vi "Joystick 1 Button Handler.vi"(8 "error in (no error)":errorcluster, 11 "Buttons":bool[](array[boolean])) -> (0 "error out":errorcluster)   [LabVIEW 2015]
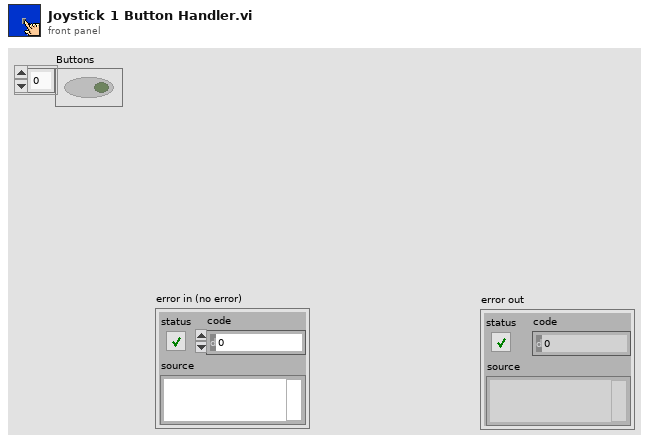
[diagram p1: front panel]
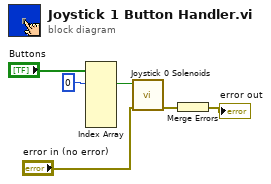
[diagram p0: block diagram]
diagram:
  n1 = Index Array(array="Buttons", index #1=0 ("index")) -> (element #1=w1:bool)  [unwired: 5 in, 5 out]
  n2 = call "Joystick 0 Solenoids.vi"("error in (no error)"="error in (no error)", "button value"=w1) -> ("error out"=w2:errorcluster)  [unwired: 9 in]
  n3 = Merge Errors(w2) -> (→"error out":errorcluster)
